vi "Radar chart ex.vi"() -> ()   [LabVIEW 2009]
panel:
  in  "X scale Range":dbl=2.0
  in  "stop":bool
  out "Triangle":dynamicdata(graph)
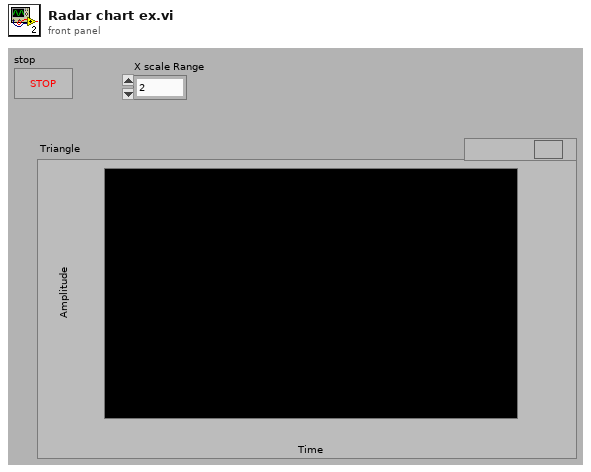
[diagram p1: front panel]
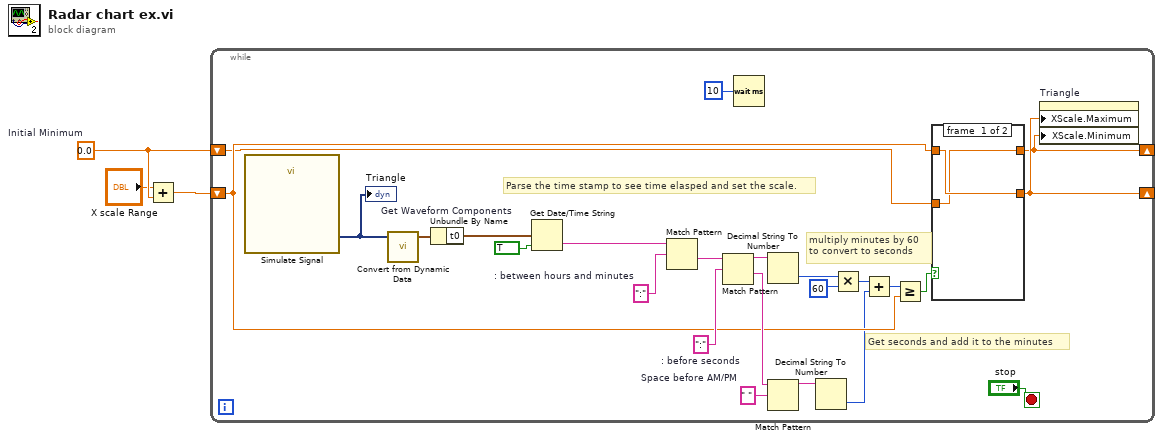
[diagram p0: block diagram]
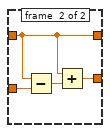
[diagram p2: hidden frame]
diagram:
  w3 = 0.0  # Initial Minimum
  n1 = Add(x="X scale Range", y=w3) -> (x+y=w1:dbl)
  n2 = while {
    shift-right: [w12] -> _
    shift-left: w1 -> [w14]
    shift-right: [w11] -> _
    shift-left: w3 -> [w13]
    stop <- "stop" stop-if-true
    w17 = " "  # Space before AM/PM
    w20 = ":"  # : before seconds
    w21 = ":"  # : between hours and minutes
    # "Get seconds and add it to the minutes"
    # "multiply minutes by 60\nto convert to seconds"
    # "Parse the time stamp to see time elasped and set the scale."
    n3 = call "Simulate Signal"() -> ("Triangle"=w26:dynamicdata)  [unwired: 14 in, 1 out]
    "Triangle" <- w26
    n4 = call "Convert from Dynamic Data"("Dynamic Data Type"=w26) -> ("Waveform"=w25:waveform(dbl))  [unwired: 3 in]
    n5 = Unbundle By Name "Get Waveform Components"(w25) -> ("t0"=w24:timestamp)
    n6 = Get Date/Time String(seconds (now)=w24, want seconds? (F)=TRUE) -> (time string=w22:string)  [unwired: 1 in, 1 out]
    n7 = Match Pattern(string=w22, regular expression=w21) -> (after substring=w19:string)  [unwired: 1 in, 3 out]
    n8 = Match Pattern(string=w19, regular expression=w20) -> (before substring=w9:string, after substring=w18:string)  [unwired: 1 in, 2 out]
    n9 = Wait (ms)(milliseconds to wait=u32 10) -> ()  [unwired: 1 out]
    n10 = Decimal String To Number(string=w9) -> (number=w8:i32)  [unwired: 2 in, 1 out]
    n11 = Match Pattern(string=w18, regular expression=w17) -> (before substring=w16:string)  [unwired: 1 in, 3 out]
    n12 = Decimal String To Number(string=w16) -> (number=w5:i32)  [unwired: 2 in, 1 out]
    n13 = Multiply(x=w8, y=60) -> (x*y=w6:i32)
    n14 = Add(x=w6, y=w5) -> (x+y=w4:i32)
    n15 = Greater Or Equal?(x=w4, y=w14) -> (x >= y?=w15:bool)
    n16 = case shown="True" w15 {
      tunnel: w14 -> [w29 w31]
      tunnel: [w29 w30] -> w12
      tunnel: w13 -> [w28 w33]
      tunnel: [w28 w31] -> w11
      frame #0 {
      }
      frame #1 {
        n17 = Subtract(x=w31, y=w33) -> (x-y=w32:dbl)
        n18 = Add(x=w31, y=w32) -> (x+y=w30:dbl)
      }
    }
    n19 = property on="Triangle" class="WFGraph (strict)"("XScale.Maximum"=w12, "XScale.Minimum"=w11) -> ()  [unwired: 2 in, 2 out]
  }
